vi "例4-4.vi"() -> ()   [LabVIEW 2019]
panel:
  out "N":dbl
  out "平方和":dbl
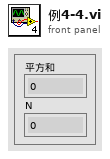
[diagram p1: front panel]
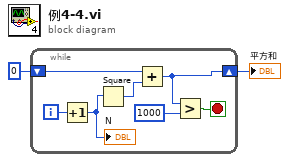
[diagram p0: block diagram]
diagram:
  n1 = while {
    shift-right: [w5] -> w1
    shift-left: 0 -> [w7]
    i -> [w9]
    stop <- w6 stop-if-true
    n2 = Increment(x=w9) -> (x+1=w3:i32)
    "N" <- w3
    n3 = Square(x=w3) -> (x^2=w8:i32)
    n4 = Add(x=w7, y=w8) -> (x+y=w5:i32)
    n5 = Greater?(x=w5, y=1000) -> (0:w6:bool)
  }
  "平方和" <- w1
